vi "ABR-Insert Notes.vi"(0 "path":path, 7 "Notes":string, 11 "error in (no error)":errorcluster) -> (4 "path out":path, 15 "error out":errorcluster)   [LabVIEW 2020]
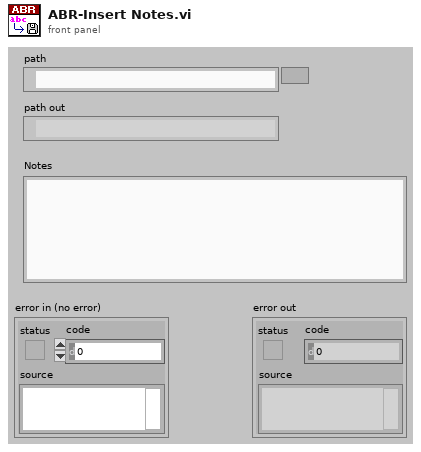
[diagram p1: front panel]
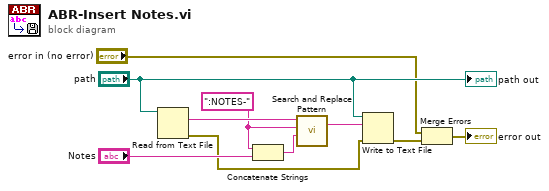
[diagram p0: block diagram]
diagram:
  w9 = ":NOTES-" ("regular expression (\"\")")
  n1 = Read from Text File(file (use dialog)="path") -> (text=w10:string, error out=w5:errorcluster)  [unwired: 3 in, 2 out]
  n2 = Concatenate Strings(w9, "Notes") -> (w7:string)
  n3 = call <vilib>:"Search and Replace Pattern.vi"("string"=w10, "regular expression (\"\")"=w9, "replace string (\"\")"=w7) -> ("result string"=w6:string)  [unwired: 2 in, 1 out]
  n4 = Write to Text File(file (use dialog)="path", text=w6, error in=w5) -> (error out=w4:errorcluster)  [unwired: 1 in, 2 out]
  n5 = Merge Errors("error in (no error)", w4) -> (→"error out":errorcluster)
  "path out" <- "path"
